vi "read_new_Flash.vi"(1 "address (3 bytes)":u32, 2 "read_bytes":u64=1) -> (0 "Read_data":u8[](array[numeric]) format="%x")   [LabVIEW 2022 SP3]
panel:
  out "InputReport1":u8[](array[numeric]) format="%x"
  out "Output Report":u8[](array[numeric])
  out "Input Report":u8[](array[numeric])
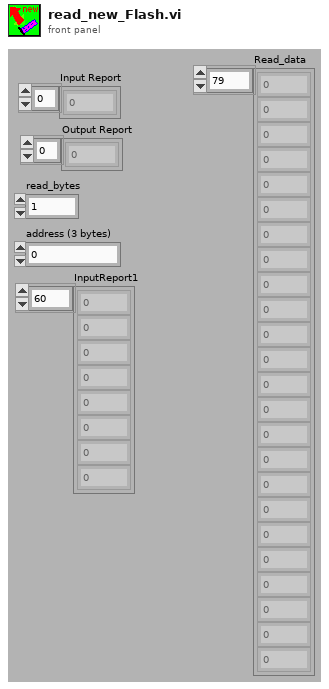
[diagram p1: front panel]
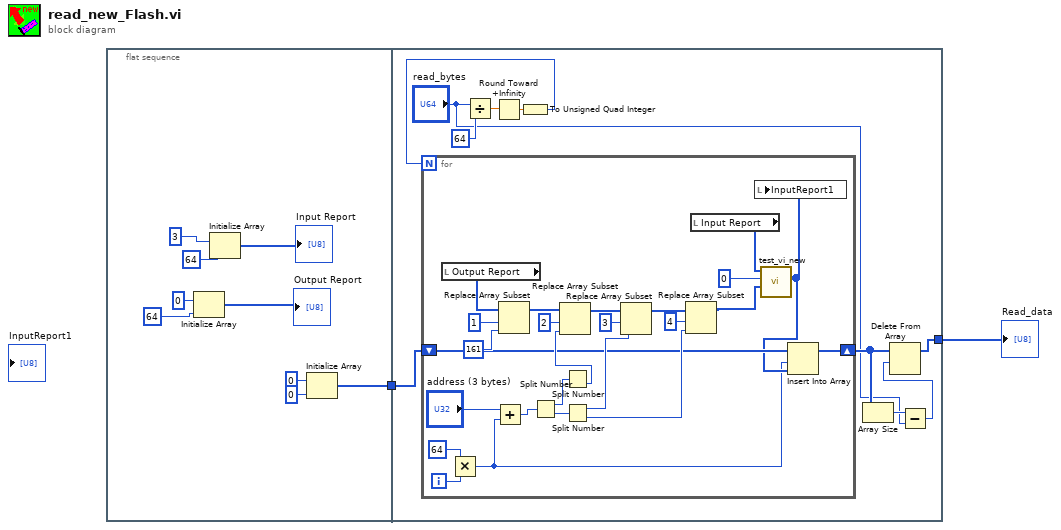
[diagram p0: block diagram]
diagram:
  n1 = flat-sequence {
    tunnel: [w3] -> w2
    tunnel: w2 -> [w17]
    tunnel: [w16] -> w1
    frame #0 {
      n2 = Initialize Array(u8 0 ("element"), 64 ("dimension size")) -> (→"Output Report":u8[])
      n3 = Initialize Array(u8 3 ("element"), 64 ("dimension size")) -> (→"Input Report":u8[])
      n4 = Initialize Array(u8 0 ("element"), 0 ("dimension size")) -> (w3:u8[])
    }
    frame #1 {
      n5 = Divide(x="read_bytes", y=64) -> (x/y=w20:dbl)
      n6 = Round Toward +Infinity(x=w20) -> (ceil(x): smallest int >= x=w19:dbl)
      n7 = To Unsigned Quad Integer(1:w19) -> (0:w18:u64)
      n8 = for {
        N: w18 -> [_]
        shift-right: [w24] -> w15
        shift-left: w17 -> [w25]
        i -> [w29]
        n9 = local read "Output Report"() -> (w43:u8[])
        n10 = Multiply(x=64, y=w29) -> (x*y=w22:i32)
        n11 = Add(x="address (3 bytes)", y=w22) -> (x+y=w26:u32)
        n12 = Replace Array Subset(array=w43, new element=u8 161 ("new element/subarray"), index=1) -> (w39:u8[])
        n13 = Split Number(x=w26) -> (hi(x)=w41:u16, lo(x)=w40:u16)
        n14 = Split Number(x=w41) -> (lo(x)=w38:u8)  [unwired: 1 out]
        n15 = Replace Array Subset(array=w39, new element=w38, index=2) -> (w36:u8[])
        n16 = Split Number(x=w40) -> (hi(x)=w35:u8, lo(x)=w32:u8)
        n17 = Replace Array Subset(array=w36, new element=w35, index=3) -> (w33:u8[])
        n18 = Replace Array Subset(array=w33, new element=w32, index=4) -> (w30:u8[])
        n19 = local read "Input Report"() -> (w42:u8[])
        n20 = call "test_vi_new.vi"("OutputReport_in"=w30, "DevDet_in"=0, "InputReport_in"=w42) -> ("InputReport_out"=w23:u8[])  [unwired: 1 in, 3 out]
        n21 = local write "InputReport1"(w23) -> ()
        n22 = Insert Into Array(array=w25, index=w22, new element=w23) -> (w24:u8[])
      }
      n23 = Array Size(array=w15) -> (size(s)=w14:i32)
      n24 = Subtract(x=w14, y="read_bytes") -> (x-y=w12:u64)
      n25 = Delete From Array(array=w15, length=w12) -> (array with subset deleted=w16:u8[])  [unwired: 1 in, 1 out]
    }
  }
  "Read_data" <- w1
